vi "EVT Get Gen I Cam Xml.vi"(10 "xml":string, 11 "camera":u64) -> (3 "function return":u32(ring))   [LabVIEW 2019, in "EmergentCameraC.lvlib"]
doc: "EMERGENTCAMERAC_API EVT_ERROR EVT_GetGenICamXml(Camera_Handle camera, const char** xml);"
uses:
  EmergentCameraC.lvlib
  emergentInstall_Windows/win64/eSDK/bin/EmergentCameraC.dll
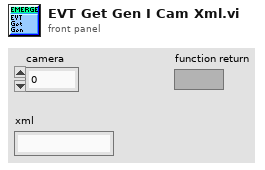
[diagram p1: front panel]
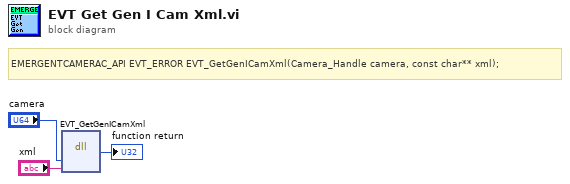
[diagram p0: block diagram]
diagram:
  # "EMERGENTCAMERAC_API EVT_ERROR EVT_GetGenICamXml(Camera_Handle camera, const char** xml);"
  n1 = dll-call lib="E:/emergent/host-new_QT/emergentInstall_Windows/win64/eSDK/bin/EmergentCameraC.*" fn="EVT_GetGenICamXml"("camera"="camera", "xml"="xml") -> (→"function return":u32)  [unwired: 5 in, 2 out]
